vi "_autosizeCluster_V.vi"(6 "Variant in":variant, 8 "error in (no error)":errorcluster, 9 "Shift Pressed?":bool, 10 "QD Combo Box Ref":refnum<vi>, 11 "QD Launch VI Ref":refnum<vi>) -> (0 "error out":errorcluster, 4 "Variant out":variant)   [LabVIEW 2014, in "NEVSTOP QD Shortcuts.lvlib"]
uses:
  NEVSTOP QD Shortcuts.lvlib
panel:
  # "Do not change the connector pane of this VI.\n\nSee the block diagram for directions on how to use this template."
  # "Specify the name of the Undo transaction"
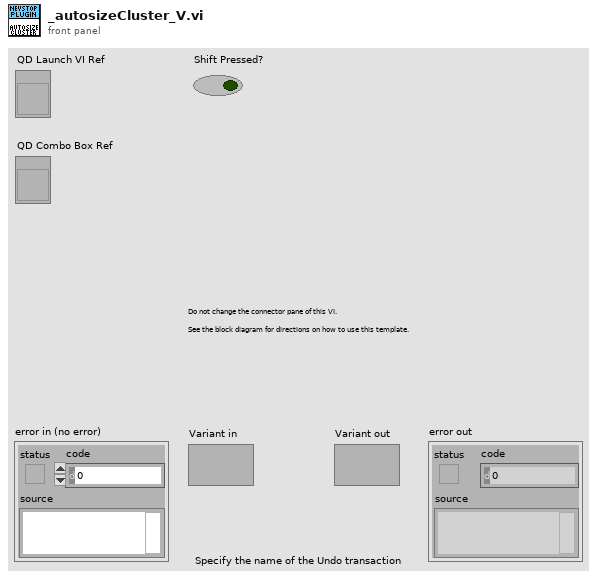
[diagram p1: front panel]
types:
  T1 = enum32{"None", "Size to Fit", "Arrange Horizontally", "Arrange Vertically"}
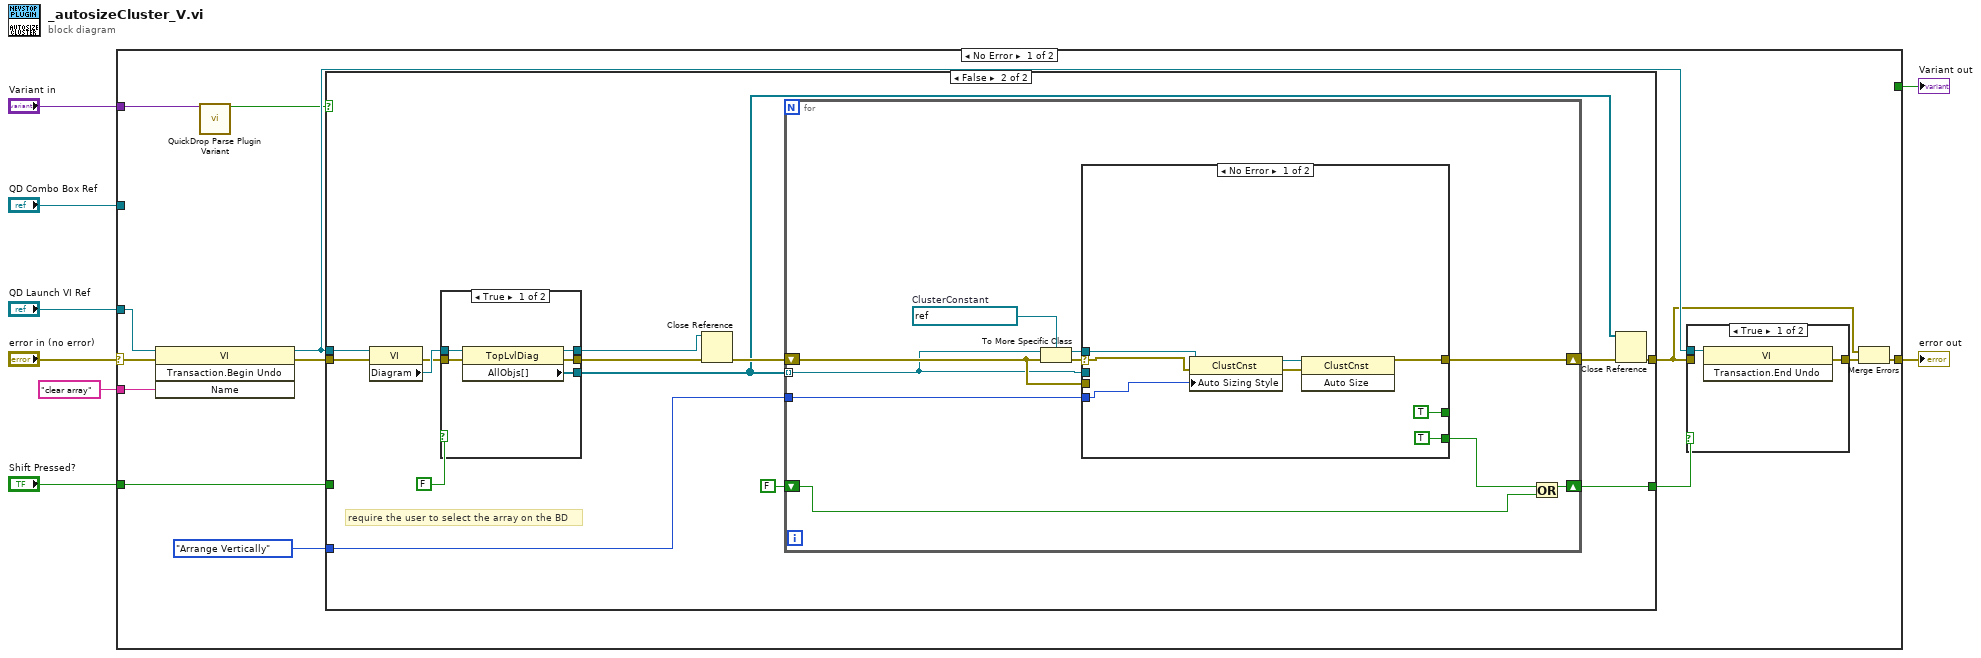
[diagram p0: block diagram]
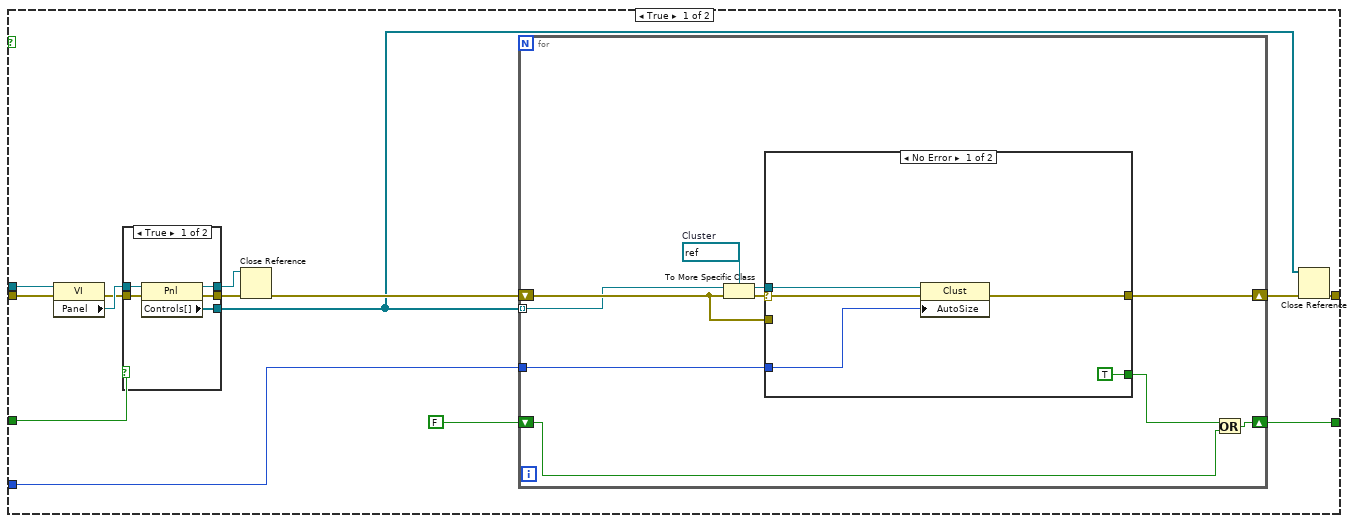
[diagram p2: hidden frame]
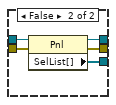
[diagram p3: hidden frame]
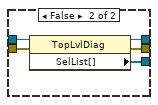
[diagram p5: hidden frame]
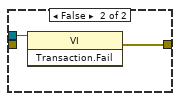
[diagram p7: hidden frame]
diagram:
  n1 = case shown="No Error" "error in (no error)" {
    selector: "error in (no error)" -> [w21 w110]
    tunnel: [w11 w110] -> w7
    tunnel: "QD Launch VI Ref" -> [w20 _]
    tunnel: "Shift Pressed?" -> [w15 _]
    tunnel: "QD Combo Box Ref" -> [_ _]
    tunnel: "Variant in" -> [w22 _]
    tunnel: "clear array" ("Undo Name") -> [w19 _]
    tunnel: [TRUE _] -> w1
    frame No Error {
      n2 = invoke class="VI" method="Transaction.Begin Undo"(reference=w20, error in=w21, "Name"=w19) -> (reference out=w14:refnum<vi>, error out=w17:errorcluster)  [unwired: 1 in, 2 out]
      n3 = call <vilib>:"QuickDrop Parse Plugin Variant.vi"("QDKS Variant in"=w22) -> ("QD Launch VI Panel?"=w13:bool)  [unwired: 12 in, 2 out]
      n4 = case shown="False" w13 {
        tunnel: w17 -> [w36 w76]
        tunnel: [w32 w73] -> w10
        tunnel: w15 -> [w27 _]
        tunnel: w14 -> [w30 w71]
        tunnel: [w25 w67] -> w12
        tunnel: T1."Arrange Vertically" ("Auto Sizing Style") -> [w23 w63]
        frame True {
          n5 = property class="VI"(reference=w30, error in=w36) -> (error out=w28:errorcluster, "Panel"=w29:refnum<vi>)  [unwired: 1 out]
          n6 = case shown="True" w27 {
            tunnel: [w41 w46] -> w34
            tunnel: [w40 w45] -> w33
            tunnel: [w39 w44] -> w31
            tunnel: w29 -> [w38 w43]
            tunnel: w28 -> [w37 w42]
            frame True {
              n7 = property class="Pnl"(reference=w38, error in=w37) -> (reference out=w40:refnum<vi>, error out=w41:errorcluster, "Controls[]"=w39:refnum<vi>[])
            }
            frame False {
              n8 = property class="Pnl"(reference=w43, error in=w42) -> (reference out=w45:refnum<vi>, error out=w46:errorcluster, "SelList[]"=w44:refnum<vi>[])
            }
          }
          n9 = Close Reference(reference=w33, error in (no error)=w34) -> (error out=w35:errorcluster)
          n10 = for {
            shift-right: [w56] -> w26
            shift-left: w35 -> [w55]
            tunnel: w31 -> [w54] mode=indexing
            shift-right: [w52] -> w25
            shift-left: FALSE -> [w51]
            tunnel: w23 -> [w50]
            w47 = refnum<vi> refnum  # Cluster
            n11 = To More Specific Class(target class=w47, reference=w54, error in=w55) -> (specific class reference=w49:refnum<vi>, error out=w48:errorcluster)
            n12 = case shown="No Error" w48 {
              selector: w48 -> [w61 _]
              tunnel: [w59 w62] -> w56
              tunnel: w49 -> [w60 _]
              tunnel: w55 -> [_ w62]
              tunnel: [TRUE _] -> w53
              tunnel: w50 -> [w57 _]
              frame No Error {
                n13 = property class="Clust"(reference=w60, error in=w61, "AutoSize"=w57) -> (error out=w59:errorcluster)  [unwired: 1 out]
              }
              frame Error {
              }
            }
            n14 = Or(x=w53, y=w51) -> (x .or. y?=w52:bool)
          }
          n15 = Close Reference(reference=w31, error in (no error)=w26) -> (error out=w32:errorcluster)
        }
        frame False {
          # "require the user to select the array on the BD"
          n16 = property class="VI"(reference=w71, error in=w76) -> (error out=w69:errorcluster, "Diagram"=w70:refnum<vi>)  [unwired: 1 out]
          n17 = case shown="True" FALSE {
            tunnel: [w81 w86] -> w74
            tunnel: [w80 w85] -> w64
            tunnel: [w79 w84] -> w72
            tunnel: w70 -> [w78 w83]
            tunnel: w69 -> [w77 w82]
            frame True {
              n18 = property class="TopLvlDiag"(reference=w78, error in=w77) -> (reference out=w80:refnum<vi>, error out=w81:errorcluster, "AllObjs[]"=w79:refnum<vi>[])
            }
            frame False {
              n19 = property class="TopLvlDiag"(reference=w83, error in=w82) -> (reference out=w85:refnum<vi>, error out=w86:errorcluster, "SelList[]"=w84:refnum<vi>[])
            }
          }
          n20 = Close Reference(reference=w64, error in (no error)=w74) -> (error out=w75:errorcluster)
          n21 = for {
            shift-right: [w96] -> w68
            shift-left: w75 -> [w95]
            tunnel: w72 -> [w91] mode=indexing
            shift-right: [w93] -> w67
            shift-left: FALSE -> [w92]
            tunnel: w63 -> [w90]
            w87 = refnum<vi> refnum  # ClusterConstant
            n22 = To More Specific Class(target class=w87, reference=w91, error in=w95) -> (specific class reference=w89:refnum<vi>, error out=w88:errorcluster)
            n23 = case shown="No Error" w88 {
              selector: w88 -> [w104 _]
              tunnel: [w98 w105] -> w96
              tunnel: w89 -> [w103 _]
              tunnel: w95 -> [_ w105]
              tunnel: [TRUE _] -> w94
              tunnel: w91 -> [_ _]
              tunnel: [TRUE _] -> _
              tunnel: w90 -> [w99 _]
              frame No Error {
                n24 = property class="ClustCnst"(reference=w103, error in=w104, "Auto Sizing Style"=w99) -> (reference out=w97:refnum<vi>, error out=w102:errorcluster)
                n25 = invoke class="ClustCnst" method="Auto Size"(reference=w97, error in=w102) -> (error out=w98:errorcluster)  [unwired: 1 in, 2 out]
              }
              frame Error {
              }
            }
            n26 = Or(x=w94, y=w92) -> (x .or. y?=w93:bool)
          }
          n27 = Close Reference(reference=w72, error in (no error)=w68) -> (error out=w73:errorcluster)
        }
      }
      n28 = case shown="True" w12 {
        tunnel: w14 -> [w106 w108]
        tunnel: [w107 w109] -> w16
        tunnel: w10 -> [_ _]
        frame True {
          n29 = invoke class="VI" method="Transaction.End Undo"(reference=w106) -> (error out=w107:errorcluster)  [unwired: 2 in, 2 out]
        }
        frame False {
          n30 = invoke class="VI" method="Transaction.Fail"(reference=w108) -> (error out=w109:errorcluster)  [unwired: 2 in, 2 out]
        }
      }
      n31 = Merge Errors(w10, w16) -> (w11:errorcluster)
    }
    frame Error {
    }
  }
  "error out" <- w7
  "Variant out" <- w1
